vi "Check_Inverter_Ready_VI.vi"() -> ()   [LabVIEW 2017]
uses:
  <vilib>/Plasmionique/MB Master/MB_Master_TCP/MB_Master_TCP.lvclass
  C:/Program Files (x86)/National Instruments/LabVIEW 2017/vi.lib/Plasmionique/MB Master/MB_Master/MB_Master.lvclass
  <vilib>/Plasmionique/MB Master/MB Master.lvlib
panel:
  out "Error?":string
  out "BMS IP Address":string
  out "Inverter IP Address":string
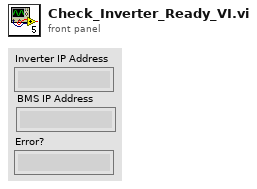
[diagram p1: front panel]
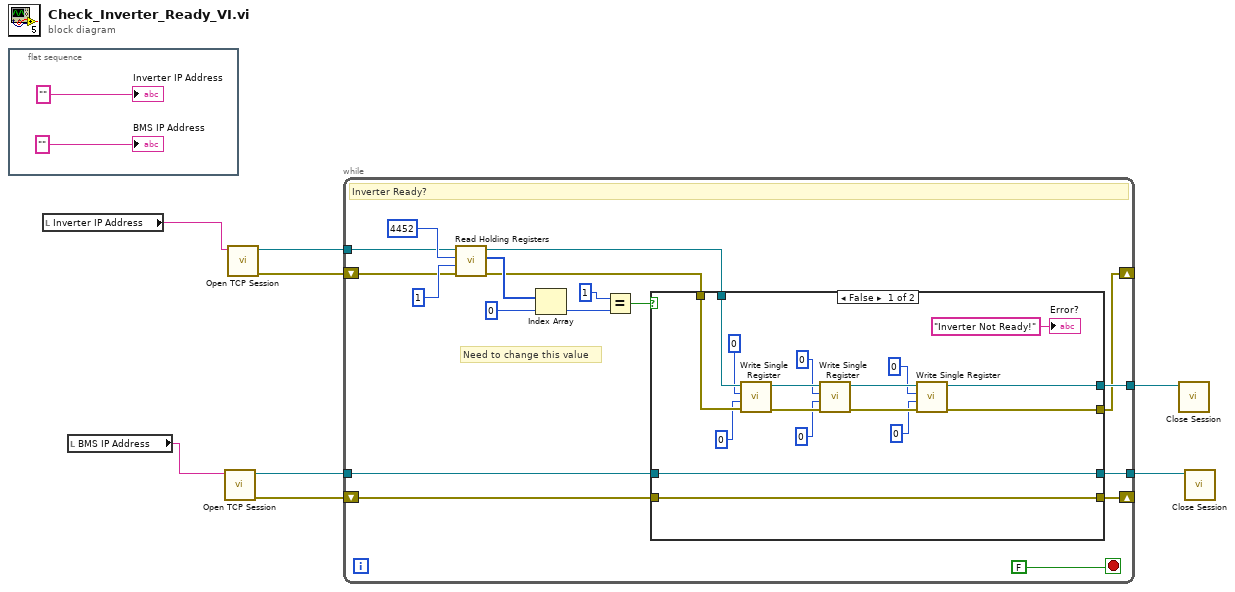
[diagram p0: block diagram]
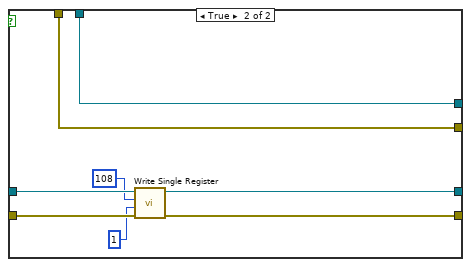
[diagram p2: hidden frame]
diagram:
  n1 = flat-sequence {
    frame #0 {
      "Inverter IP Address" <- "" ("Inverter IP Address")
      "BMS IP Address" <- "" ("String")
    }
  }
  n2 = local read "Inverter IP Address"() -> (w8:string)
  n3 = local read "BMS IP Address"() -> (w5:string)
  n4 = call <vilib>:"Open TCP Session.vi"("IP Address"=w5) -> ("error out"=w3:errorcluster, "MB_TCP session"=w4:refnum<class "MB_Master_TCP.lvclass">)  [unwired: 9 in]
  n5 = call <vilib>:"Open TCP Session.vi"("IP Address"=w8) -> ("error out"=w7:errorcluster, "MB_TCP session"=w6:refnum<class "MB_Master_TCP.lvclass">)  [unwired: 9 in]
  n6 = while {
    tunnel: w6 -> [w21]
    tunnel: w4 -> [w18]
    tunnel: [w16] -> w2
    tunnel: [w12] -> w1
    shift-right: [w15] -> _
    shift-left: w3 -> [w17]
    shift-right: [w11] -> _
    shift-left: w7 -> [w20]
    stop <- FALSE stop-if-true
    # "Need to change this value"
    # "Inverter Ready?"
    n7 = call <vilib>:"Read Holding Registers.vi"("error in (no error)"=w20, "quantity"=u16 1, "starting address"=u16 4452, "MB session in"=w21) -> ("error out"=w13:errorcluster, "Registers"=w25:u16[], "MB session out"=w14:refnum<class "MB_Master_TCP.lvclass">)  [unwired: 5 in]
    n8 = Index Array(array=w25, index=0) -> (element=w23:u16)
    n9 = Equal?(x=u16 1, y=w23) -> (x = y?=w19:bool)
    n10 = case shown="False" w19 {
      tunnel: w18 -> [w44 w53]
      tunnel: w17 -> [w43 w52]
      tunnel: [w44 w49] -> w16
      tunnel: [w43 w48] -> w15
      tunnel: w14 -> [w41 w46]
      tunnel: w13 -> [w42 w47]
      tunnel: [w36 w46] -> w12
      tunnel: [w35 w47] -> w11
      frame False {
        n11 = call <vilib>:"Write Single Register.vi"("error in (no error)"=w42, "value"=u16 0, "address"=u16 0, "MB session in"=w41) -> ("error out"=w38:errorcluster, "MB session out"=w40:refnum<class "MB_Master_TCP.lvclass">)  [unwired: 6 in]
        n12 = call <vilib>:"Write Single Register.vi"("error in (no error)"=w38, "value"=u16 0, "address"=u16 0, "MB session in"=w40) -> ("error out"=w37:errorcluster, "MB session out"=w39:refnum<class "MB_Master_TCP.lvclass">)  [unwired: 6 in]
        n13 = call <vilib>:"Write Single Register.vi"("error in (no error)"=w37, "value"=u16 0, "address"=u16 0, "MB session in"=w39) -> ("error out"=w35:errorcluster, "MB session out"=w36:refnum<class "MB_Master_TCP.lvclass">)  [unwired: 6 in]
        "Error?" <- "Inverter Not Ready!" ("Error?")
      }
      frame True {
        n14 = call <vilib>:"Write Single Register.vi"("error in (no error)"=w52, "value"=u16 1, "address"=u16 108, "MB session in"=w53) -> ("error out"=w48:errorcluster, "MB session out"=w49:refnum<class "MB_Master_TCP.lvclass">)  [unwired: 6 in]
      }
    }
  }
  n15 = call-dynamic "Close Session.vi"("MB TCP session"=w1) -> ()  [unwired: 10 in, 1 out]
  n16 = call-dynamic "Close Session.vi"("MB TCP session"=w2) -> ()  [unwired: 10 in, 1 out]
